vi "MaxTimeoutWatchdog.vi"(10 "Keep counting?":bool, 11 "Max Timeout (s)":dbl) -> (3 "Over Max Timeout?":bool)   [LabVIEW 2017, in "Subsystem.lvclass"]
uses:
  Subsystem.lvclass
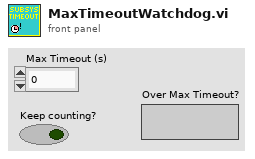
[diagram p1: front panel]
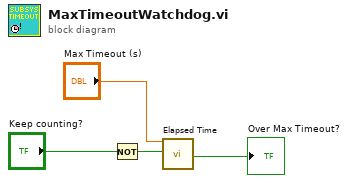
[diagram p0: block diagram]
diagram:
  n1 = Not(x="Keep counting?") -> (.not. x?=w3:bool)
  n2 = call "Elapsed Time"("Time Target (s)"="Max Timeout (s)", "Reset"=w3) -> ("Time has Elapsed"=→"Over Max Timeout?":bool)  [unwired: 10 in, 7 out]
